vi "subVI moving average.vi"(2 "lenght":dbl, 3 "input":waveform(i64)) -> (0 "output":waveform(i64))   [LabVIEW 2012]
uses:
  <vilib>/Analysis/3filter.llb/FIR Filter (DBL).vi
  <vilib>/Analysis/NI_AALBase.lvlib
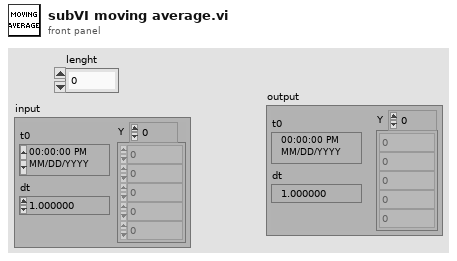
[diagram p1: front panel]
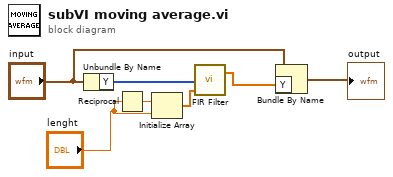
[diagram p0: block diagram]
diagram:
  n1 = Unbundle By Name("input") -> ("Y"=w5:i64[])
  n2 = Reciprocal(x="lenght") -> (1/x=w7:dbl)
  n3 = Initialize Array(w7, "lenght") -> (w6:dbl[])
  n4 = call-poly <vilib>:"FIR Filter.vi"("FIR Coefficients"=w6, "X"=w5) -> ("Filtered X"=w4:dbl[])  [unwired: 2 in, 1 out]
  n5 = Bundle By Name(cluster="input", "Y"=w4) -> (→"output":waveform(i64))
